vi "InitializeSessions.vi"(0 "NI-DMM in":refnum<class "NI-DMM.lvclass">, 5 "InitializeSessionsInfo":variant, 11 "error in":errorcluster) -> (4 "NI-DMM out":refnum<class "NI-DMM.lvclass">, 15 "error out":errorcluster)   [LabVIEW 2020, in "Abstract_Instrument.lvlib" / "NI-DMM.lvclass"]
uses:
  NI-DMM.lvclass
  TypeDef/Initialize_Information.ctl
  <vilib>/MeasurementLink/MeasurementLink Session Management V1/Session Reservation/Initialize and Close Session Behavior.ctl
  NI-DMM.lvclass/NI-DMM.ctl
  <vilib>/MeasurementLink/MeasurementLink niDMM/Initialize Sessions - 1Sess.vi
  Base/Abstract_Instrument.lvclass
  <vilib>/MeasurementLink/MeasurementLink Session Management V1/Session Reservation/Session Reservation.lvclass
  <vilib>/MeasurementLink/MeasurementLink niDMM/MeasurementLink niDMM.lvlib
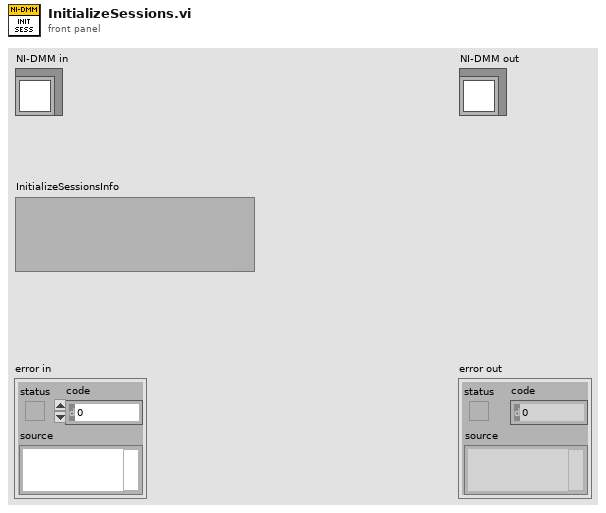
[diagram p1: front panel]
types:
  T1 = typedef "Abstract_Instrument.lvlib/NI-DMM.lvclass/Initialize_Information.ctl" = cluster{"initialize and close session behavior":T2, "reset":bool}
  T2 = typedef "MeasurementLink Session Management V1.lvlib/Session Reservation.lvclass/Initialize and Close Session Behavior.ctl" = enum16{"Auto", "Initialize and Close", "Attach and Detach", "Initialize and Detach", "Attach and Close"}
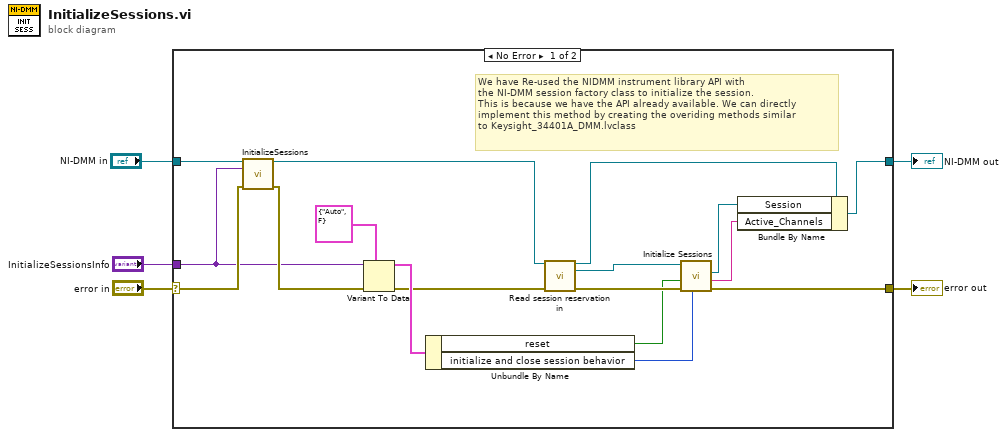
[diagram p0: block diagram]
diagram:
  n1 = case shown="No Error" "error in" {
    selector: "error in" -> [w21 w23]
    tunnel: "NI-DMM in" -> [w22 w24]
    tunnel: "InitializeSessionsInfo" -> [w19 _]
    tunnel: [w11 w23] -> w2
    tunnel: [w7 w24] -> w1
    frame No Error {
      # "We have Re-used the NIDMM instrument library API with \nthe NI-DMM session factory class to initialize the session.\nThis is because we have the API already available. We can directly\nimplement this method by creating the overiding methods similar\nto Keysight_34401A_DMM.lvclass"
      n2 = call-parent "InitializeSessions.vi"("AbstractDMM in"=w22, "InitializeSessionsInfo"=w19, "error in (no error)"=w21) -> ("AbstractDMM out"=w16:refnum<class "NI-DMM.lvclass">, "error out"=w20:errorcluster)  [unwired: 11 in]
      n3 = Variant To Data(error in=w20, type=T1 {"initialize and close session behavior"=enum."Auto", "reset"=FALSE} ("Initialize_Information"), Variant=w19) -> (data=w17:T1, error out=w15:errorcluster)
      n4 = Unbundle By Name(w17) -> ("reset"=w10:bool, "initialize and close session behavior"=w13:T2)
      n5 = call-dynamic "Read session reservation in.vi"("AbstractDMM in"=w16, "error in (no error)"=w15) -> ("AbstractDMM out"=w8:refnum<class "NI-DMM.lvclass">, "MeasurementLink Session Management V1.lvlib:Session Reservation.lvclass"=w14:refnum<class "Session Reservation.lvclass">, "error out"=w12:errorcluster)  [unwired: 11 in]
      n6 = call-poly <vilib>:"Initialize Sessions.vi"("initialize and close session behavior"=w13, "error in"=w12, "reset"=w10, "session reservation in"=w14) -> ("error out"=w11:errorcluster, "channel list"=w6:string, "session"=w9:refnum<k15>)  [unwired: 4 in, 1 out]
      n7 = Bundle By Name(cluster=w8, "Session"=w9, "Active_Channels"=w6) -> (w7:refnum<class "NI-DMM.lvclass">)
    }
    frame Error {
    }
  }
  "error out" <- w2
  "NI-DMM out" <- w1
